vi "DriveModuleControl_TravTuneKsKv.vi"(8 "error in":errorcluster, 9 "Actual State":T1={"Speed"=0.0, "Angle"={"VALUE"=0.0, "COS"=1.0, "SIN"=0.0}} {"Angle"."SIN" format="%13.4f"; "Angle"."COS" format="%13.4f"; "Angle"."VALUE" format="%13.4f"}, 10 "Desired State":T1={"Speed"=0.0, "Angle"={"VALUE"=0.0, "COS"=1.0, "SIN"=0.0}} {"Angle"."SIN" format="%13.4f"; "Angle"."COS" format="%13.4f"; "Angle"."VALUE" format="%13.4f"}, 11 "ModualNamePrefix":i32) -> (0 "error out":errorcluster)   [LabVIEW 2023]
uses:
  <vilib>/Rock Robotics/WPI/ThirdParty/JAS_Junk/TrajLib/TypeDef/SWERVE_DRIVE_MODULE_STATE.ctl
  <vilib>/Rock Robotics/WPI/ThirdParty/JAS_Junk/TrajLib/TypeDef/ROTATION2D.ctl
  <vilib>/Rock Robotics/WPI/ThirdParty/JAS_Junk/TrajLib/LinearFilter_MovingAvg_Execute.vi
  <vilib>/Rock Robotics/WPI/ThirdParty/JAS_Junk/TrajLib/Rotation2d_Minus.vi
  <vilib>/Rock Robotics/WPI/ThirdParty/JAS_Junk/TrajLib/Rotation2d_GetRadians.vi
  <vilib>/Rock Robotics/WPI/ThirdParty/JAS_Junk/TrajLib/SwerveModuleState_New.vi
  <vilib>/Rock Robotics/WPI/ThirdParty/JAS_Junk/TrajLib/Rotation2d_RotateBy.vi
  <vilib>/Rock Robotics/WPI/ThirdParty/JAS_Junk/TrajLib/Rotation2d_CreateAngle.vi
  <vilib>/Rock Robotics/WPI/ThirdParty/JAS_Junk/TrajLib/SimpleMotorFF_Calculate.vi
  <vilib>/Rock Robotics/WPI/ThirdParty/JAS_Junk/TrajLib/PIDController_AtSetpoint.vi
  <vilib>/Rock Robotics/WPI/ThirdParty/JAS_Junk/TrajLib/PIDController_SetPIDF.vi
  <vilib>/Rock Robotics/WPI/ThirdParty/JAS_Junk/TrajLib/PIDController_SetDerivativeFilter.vi
  <vilib>/Rock Robotics/WPI/ThirdParty/JAS_Junk/TrajLib/PIDController_SetIntegratorRange.vi
  <vilib>/Rock Robotics/WPI/ThirdParty/JAS_Junk/TrajLib/PIDController_SetTolerancePandV.vi
  <vilib>/Rock Robotics/WPI/ThirdParty/JAS_Junk/TrajLib/PIDController_DisableContinousInput.vi
  <vilib>/Rock Robotics/WPI/ThirdParty/JAS_Junk/TrajLib/PIDController_EnableContinousInput.vi
  <vilib>/Rock Robotics/WPI/ThirdParty/JAS_Junk/TrajLib/PIDController_Reset.vi
  <vilib>/Rock Robotics/WPI/ThirdParty/JAS_Junk/TrajLib/PIDController_New.vi
  <vilib>/Rock Robotics/WPI/ThirdParty/JAS_Junk/TrajLib/PIDController_SetOutputLimits.vi
  <vilib>/Rock Robotics/WPI/ThirdParty/JAS_Junk/TrajLib/VI/PIDController_SetIntegratorZone.vi
  <vilib>/Rock Robotics/WPI/ThirdParty/JAS_Junk/TrajLib/LinearFilter_ResetToValue.vi
  <vilib>/Rock Robotics/WPI/ThirdParty/JAS_Junk/TrajLib/LinearFilter_Calculate.vi
  <vilib>/Rock Robotics/WPI/ThirdParty/JAS_Junk/TrajLib/Rotation2d_UnaryMinus.vi
  <vilib>/Rock Robotics/WPI/ThirdParty/JAS_Junk/TrajLib/Rotation2d_CreateXY.vi
  <vilib>/Rock Robotics/WPI/ThirdParty/JAS_Junk/TrajLib/PIDController_NewPeriod.vi
  <vilib>/Rock Robotics/WPI/ThirdParty/JAS_Junk/TrajLib/Util_CalcDist.vi
  <vilib>/Rock Robotics/SystemInterfaces/NetworkCommunication/NetComm_UsageReport_report.vi
  DriveGlobal.vi
  <vilib>/Rock Robotics/WPI/ThirdParty/Phoenix6/Phoenix6_Device_RefNumRegistryGet.vi
  <vilib>/Rock Robotics/WPI/MotorControl/WPI_MotorControlRefNum Registry Get.vi
  <vilib>/Rock Robotics/Network Tables/NT Write Number.vi
  <vilib>/Rock Robotics/WPI/ThirdParty/JAS_Junk/TrajLib/LinearFilter_MovingAverage.vi
  <vilib>/Utility/semaphor.llb/Obtain Semaphore Reference.vi
  <vilib>/Rock Robotics/WPI/ThirdParty/JAS_Junk/TrajLib/Timer_Reset.vi
  DriveTuningGlobals.vi
  <vilib>/Rock Robotics/WPI/ThirdParty/JAS_Junk/TrajLib/Globals/Util_LibraryGlobals.vi
  <vilib>/Rock Robotics/WPI/ThirdParty/JAS_Junk/TrajLib/PIDController_AdvCalculate_FF_Sp_Pv.vi
  <vilib>/Rock Robotics/WPI/ThirdParty/JAS_Junk/TrajLib/Trajectory_Library.lvlib
  <vilib>/Rock Robotics/WPI/ThirdParty/REV Robotics/REVLib/Typedef/Spark MAX Control Type.ctl
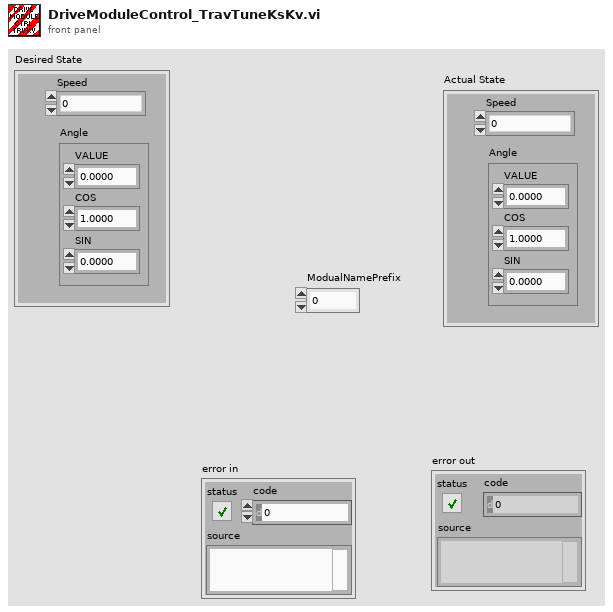
[diagram p1: front panel]
types:
  T1 = typedef "Trajectory_Library.lvlib/SWERVE_DRIVE_MODULE_STATE.ctl" = cluster{"Speed":dbl, "Angle":T2}
  T2 = typedef "Trajectory_Library.lvlib/ROTATION2D.ctl" = cluster{"VALUE":dbl, "COS":dbl, "SIN":dbl}
  T3 = typedef "Spark MAX Control Type.ctl" = enum16{"Percent VBus", "Voltage", "Velocity", "Position", "Smart Motion", "Current", "Smart Velocity", "MAXMotion Position", "MAXMotion Velocity"}
  T4 = typedef "WPI_MotorControlDeviceRef.ctl" = cluster{"DeviceStatus":errorcluster, "Type":T5, "PWM":cluster{"PWM Channel":T6, "DeadBand":T7}, "CAN":cluster{"Device Number":u8, "SetOutput VI Ref":variant, "GetOutput VI Ref":variant, "Enable VI Ref":variant, "Disable VI Ref":variant, "Data":variant}, "Invert":bool, "DIO PWM":cluster{"PWM \"Enable\" Channel":T6, "DIOChannel":T8, "PWM Rate":dbl}}
  T5 = typedef "WPI_MotorControlType.ctl" = enum16{"PWM", "CAN", "DIO PWM"}
  T6 = typedef "FPGA_DIOPWMChannel.ctl" = enum8{"PWM 0", "PWM 1", "PWM 2", "PWM 3", "PWM 4", "PWM 5", "PWM 6", "PWM 7", "PWM 8", "PWM 9", "PWM MXP 0", "PWM MXP 1", "PWM MXP 2", "PWM MXP 3", "PWM MXP 4", "PWM MXP 5", "PWM MXP 6", "PWM MXP 7", "PWM MXP 8", "PWM MXP 9", "Invalid"}
  T7 = typedef "WPI_PWMDeadband.ctl" = cluster{"Name":string, "maxPositivePwm":i32, "minPositivePwm":i32, "centerPwm":i32, "maxNegativePwm":i32, "minNegativePwm":i32, "angularRange":u16}
  T8 = typedef "FPGA_DIOChannel.ctl" = enum8{"DIO 0", "DIO 1", "DIO 2", "DIO 3", "DIO 4", "DIO 5", "DIO 6", "DIO 7", "DIO 8", "DIO 9", "DIO MXP 0", "DIO MXP 1", "DIO MXP 2", "DIO MXP 3", "DIO MXP 4", "DIO MXP 5", "DIO MXP 6", "DIO MXP 7", "DIO MXP 8", "DIO MXP 9", "DIO MXP 10", "DIO MXP 11", "DIO MXP 12", "DIO MXP 13", "DIO MXP 14", "DIO MXP 15", "SPI Port CS1", "SPI Port CS2", "SPI Port CS3", "SPI Port MISO", "SPI Port MOSI", "Invalid"}
  T9 = typedef "Trajectory_Library.lvlib/TIMER.ctl" = cluster{"StartTime":dbl, "Accumulated TIme":dbl, "Running":bool, "semaphore":T10}
  T10 = typedef "Semaphore RefNum" = refnum<k1>
  T11 = typedef "Trajectory_Library.lvlib/SIMPLE_MOTOR_FF.ctl" = cluster{"Ks":dbl, "Kv":dbl, "Ka":dbl, "KnInv":dbl}
  T12 = typedef "Trajectory_Library.lvlib/PID_ADV_LIMITS.ctl" = cluster{"MaxInput":dbl, "MinInput":dbl, "Continuous":bool, "MaxOutput":dbl, "MinOutput":dbl}
  T13 = typedef "Trajectory_Library.lvlib/PID_ADV_TUNING.ctl" = cluster{"Kf":dbl, "Kp":dbl, "Ki":dbl, "Kd":dbl, "MaximumIntegral":dbl, "MinimumIntegral":dbl, "Filter Derivative":bool, "IntegralZone":dbl}
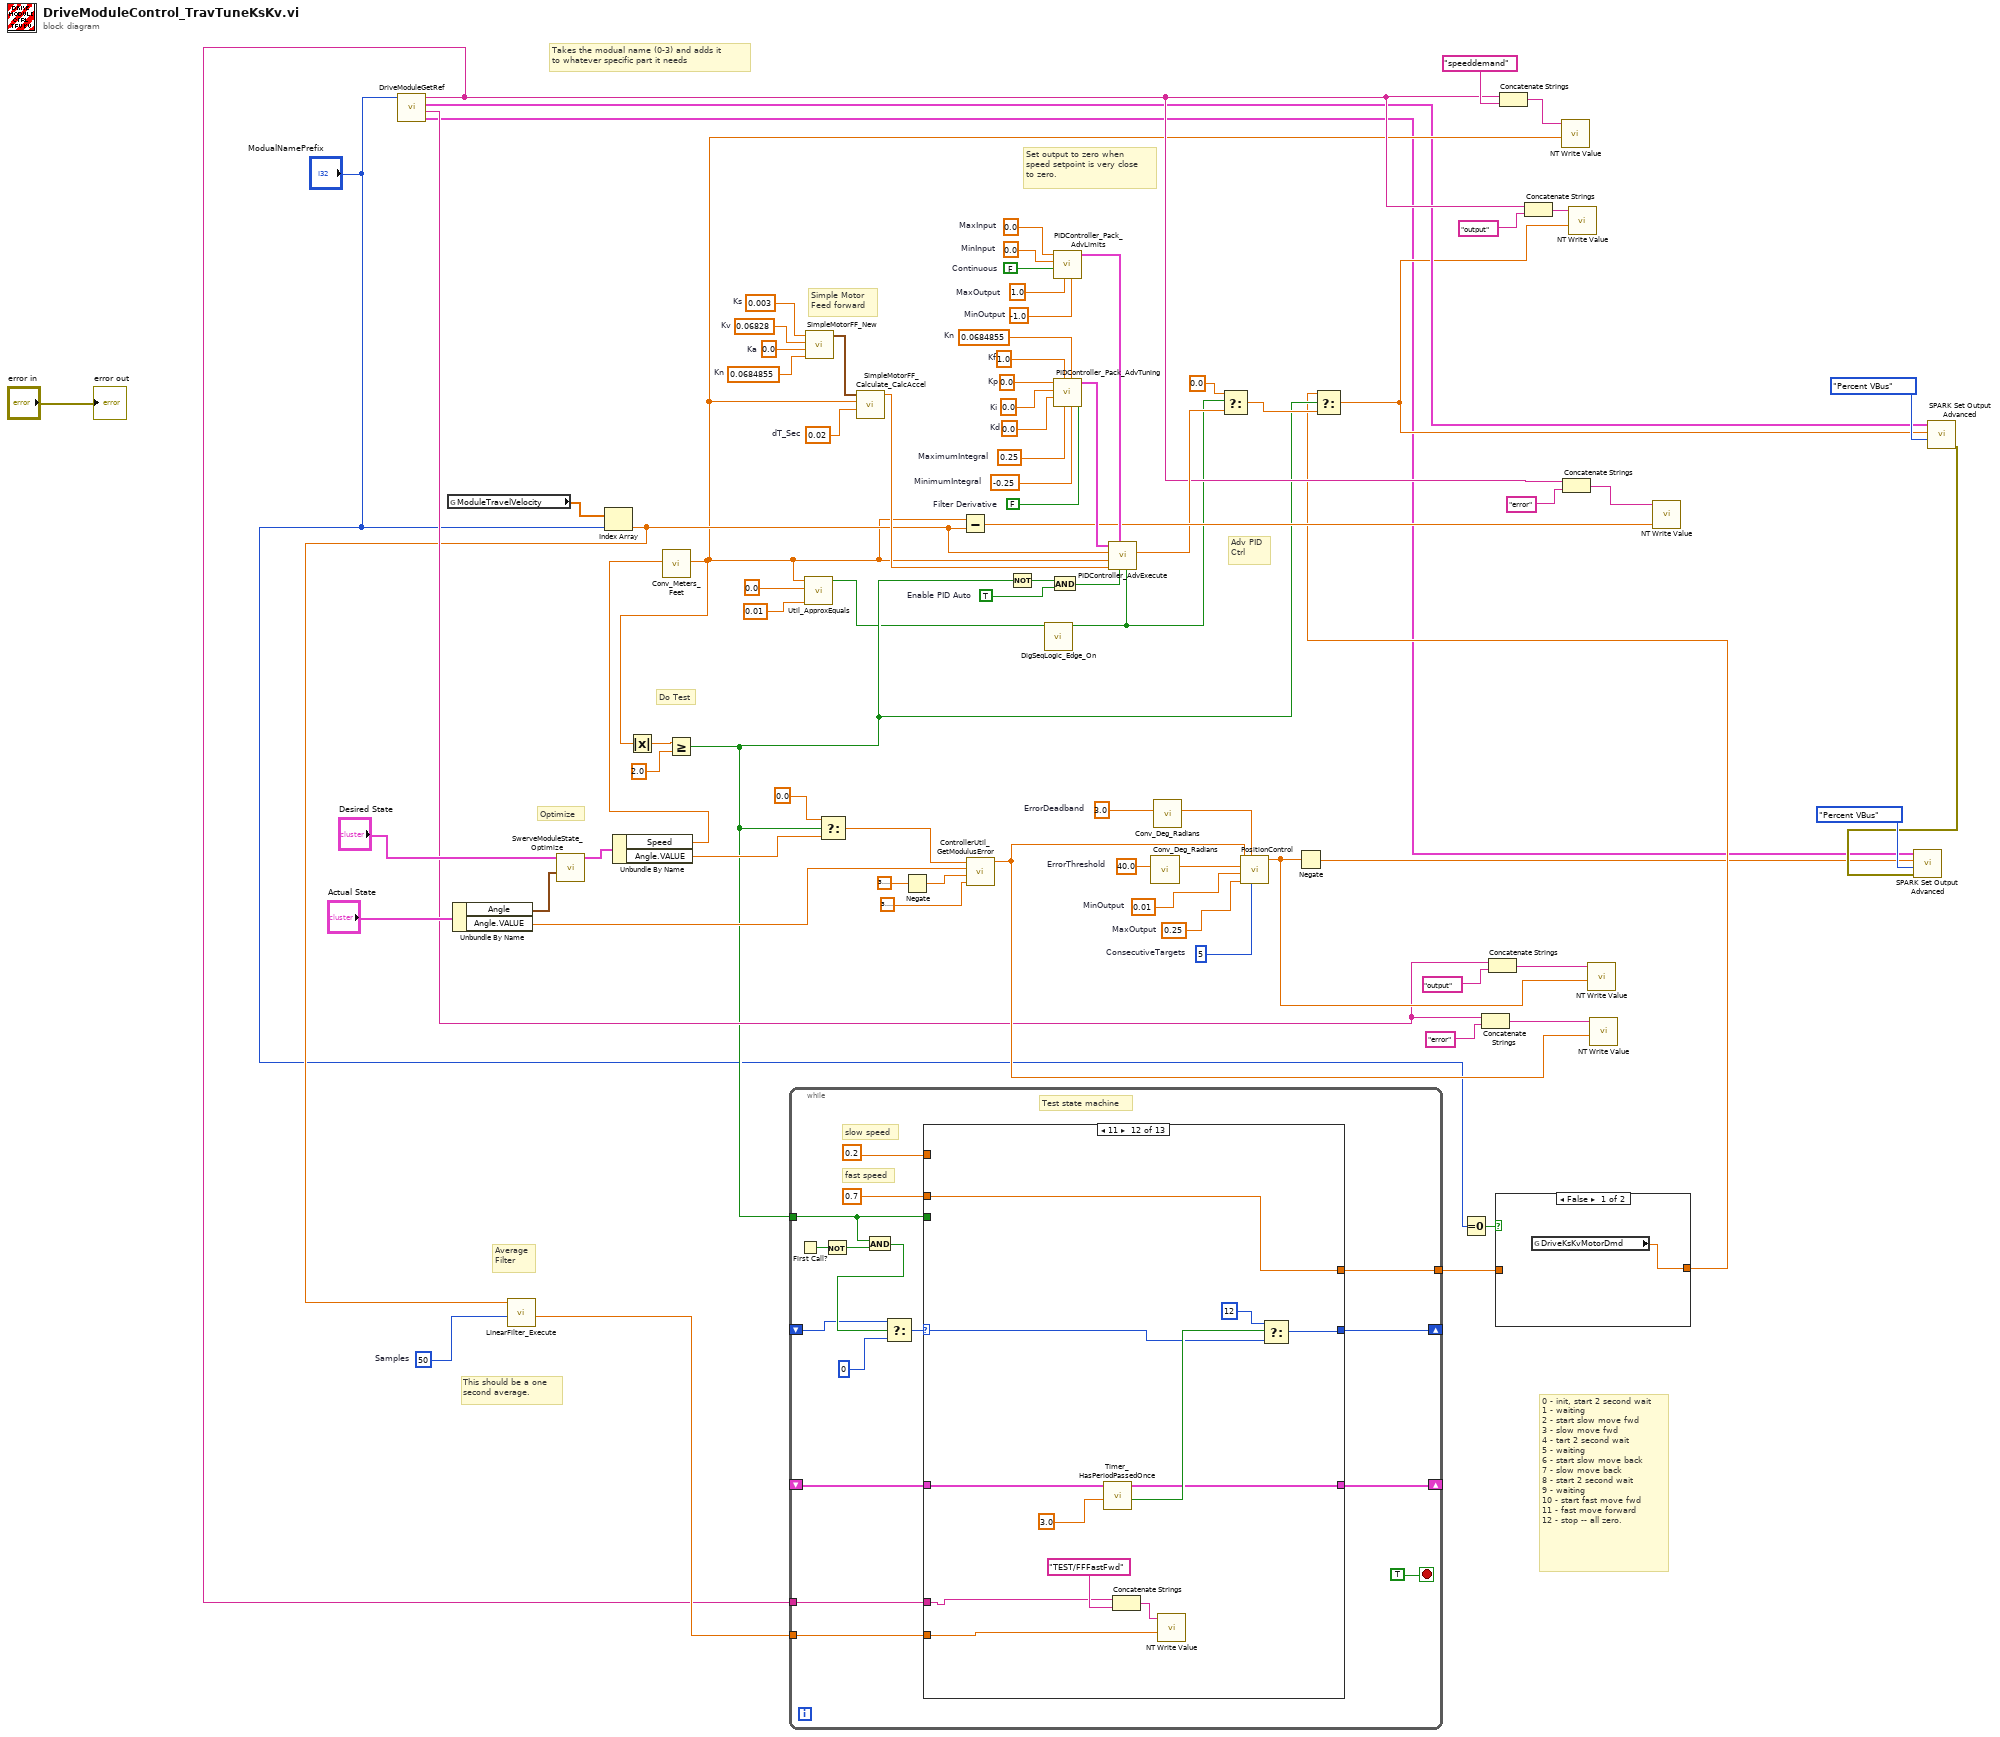
[diagram p0: block diagram]
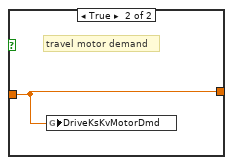
[diagram p2: hidden frame]
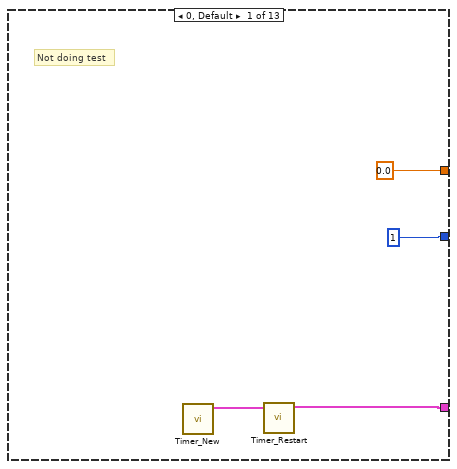
[diagram p3: hidden frame]
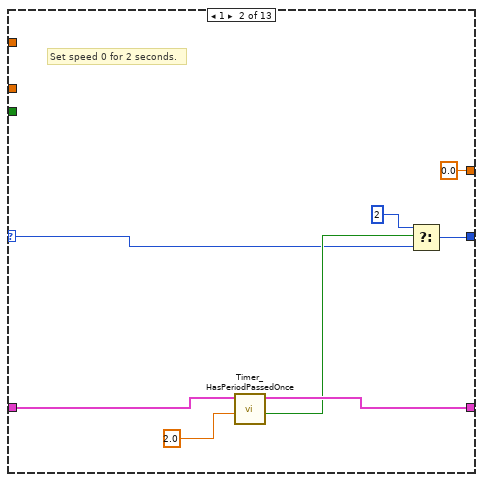
[diagram p4: hidden frame]
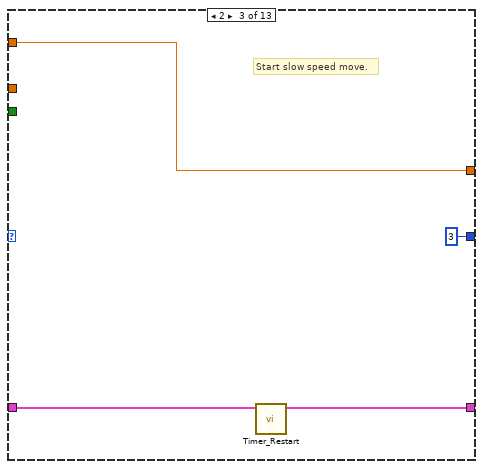
[diagram p5: hidden frame]
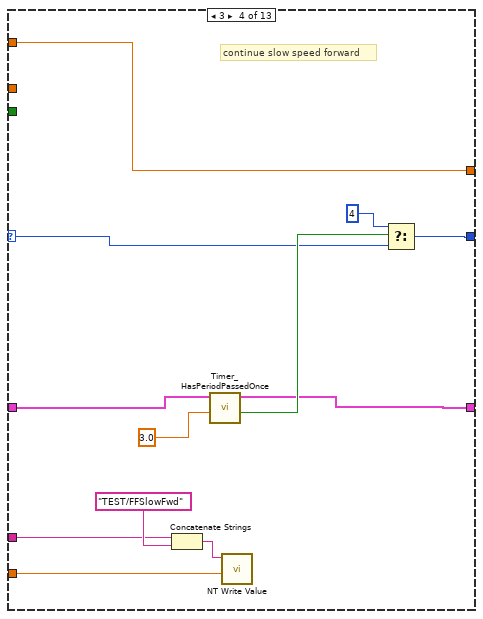
[diagram p6: hidden frame]
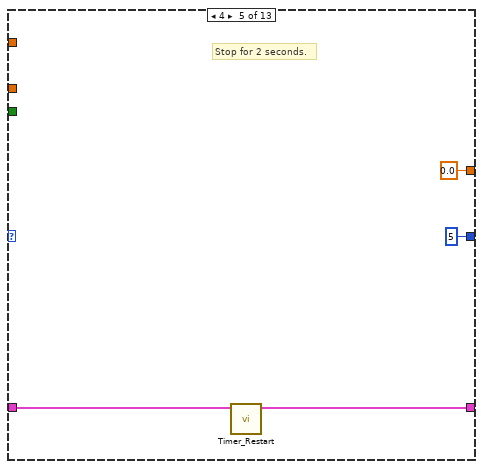
[diagram p7: hidden frame]
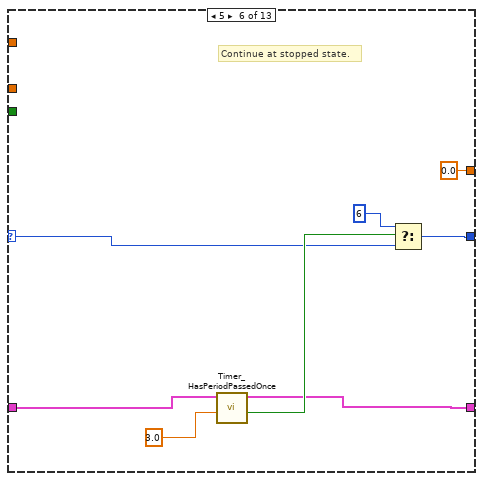
[diagram p8: hidden frame]
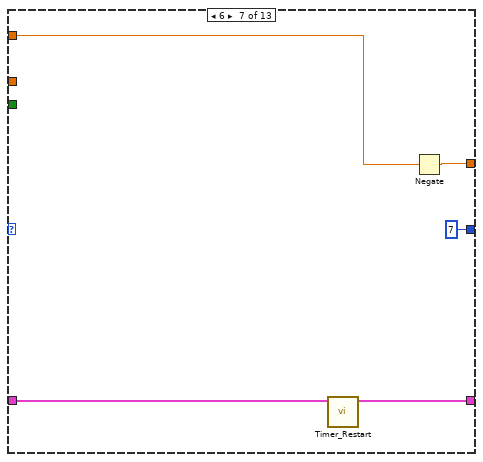
[diagram p9: hidden frame]
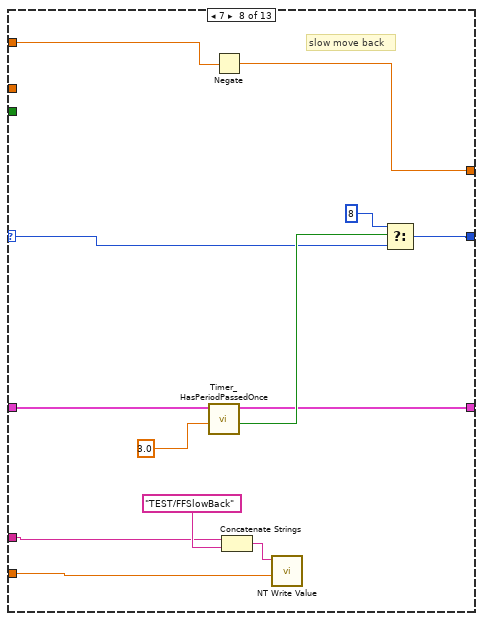
[diagram p10: hidden frame]
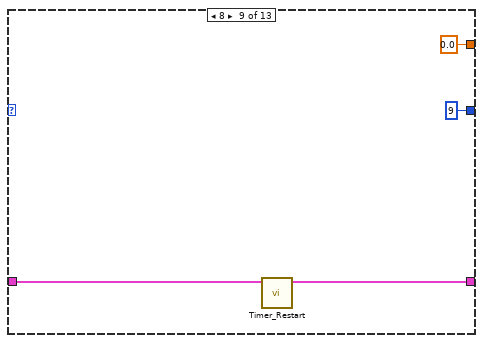
[diagram p11: hidden frame]
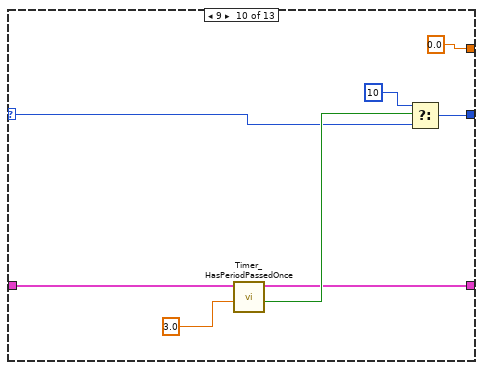
[diagram p12: hidden frame]
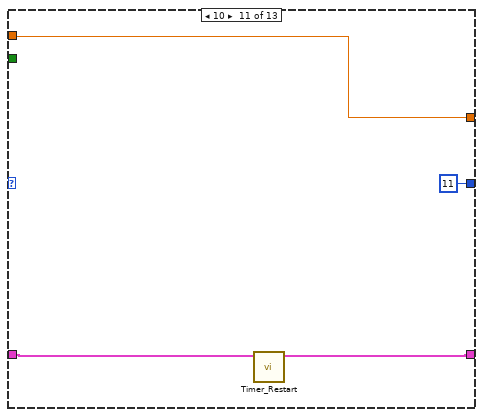
[diagram p13: hidden frame]
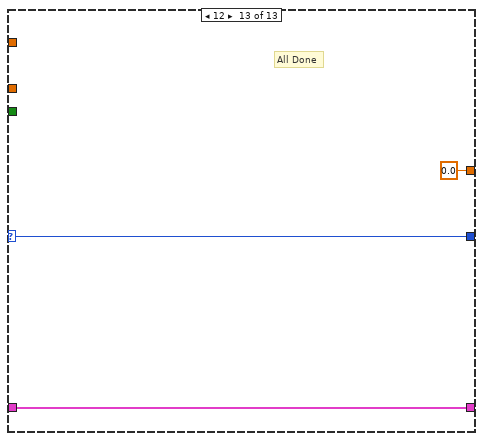
[diagram p14: hidden frame]
diagram:
  w15 = 50  # Samples
  w29 = TRUE  # Enable PID Auto
  w38 = 0.0684855  # Kn
  w54 = 0.0  # Kp
  w53 = 0.0  # Ki
  w52 = 0.0  # Kd
  w51 = 1.0  # Kf
  w50 = 0.25  # MaximumIntegral
  w49 = -0.25  # MinimumIntegral
  w48 = FALSE  # Filter Derivative
  w46 = 0.0  # MinInput
  w45 = FALSE  # Continuous
  w44 = 1.0  # MaxOutput
  w47 = -1.0  # MinOutput
  w43 = 0.0  # MaxInput
  w60 = 0.0684855  # Kn
  w59 = 0.02  # dT_Sec
  w57 = 0.003  # Ks
  w56 = 0.06828  # Kv
  w55 = 0.0  # Ka
  w69 = 5  # ConsecutiveTargets
  w66 = 0.25  # MaxOutput
  w70 = 0.01  # MinOutput
  w63 = 40.0  # ErrorThreshold
  w65 = 3.0  # ErrorDeadband
  # "This should be a one\nsecond average."
  # "Average\nFilter"
  # "0 - init, start 2 second wait\n1 - waiting\n2 - start slow move fwd\n3 - slow move fwd\n4 - tart 2 second wait\n5 - waiting\n6 - start slow move back\n7 - slow move back\n8 - start 2 second wait\n9 - waiting\n10 - start fast move fwd\n11 - fast move forward\n12 - stop -- all zero."
  # "Do Test"
  # "Optimize"
  # "Set output to zero when\nspeed setpoint is very close\nto zero."
  # "Adv PID\nCtrl"
  # "Simple Motor\nFeed forward"
  # "Takes the modual name (0-3) and adds it \nto whatever specific part it needs"
  n1 = call "DriveModuleGetRef.vi"("ModualNamePrefix"="ModualNamePrefix") -> ("SpinMot"=w2:T4, "SpinStr"=w34:string, "TravMot"=w4:T4, "TravStr"=w17:string)  [unwired: 5 in, 2 out]
  n2 = global read "DriveGlobal.vi" "ModuleTravelVelocity"() -> (w39:dbl[])
  n3 = Unbundle By Name("Actual State") -> ("Angle"=w76:T2, "Angle.VALUE"=w73:dbl)
  n4 = call <vilib>:"SwerveModuleState_Optimize.vi"("CurrentAngle"=w76, "Desired State"="Desired State") -> ("out SWERVE_DRIVE_MODULE_STATE"=w74:T1)  [unwired: 9 in]
  n5 = Index Array(array=w39, index="ModualNamePrefix") -> (element=w19:dbl)
  n6 = call-poly <vilib>:"LinearFilter_Execute.vi"("Samples"=w15, "Input"=w19) -> ("Output"=w18:dbl)  [unwired: 9 in]
  n7 = Unbundle By Name(w74) -> ("Speed"=w26:dbl, "Angle.VALUE"=w23:dbl)
  n8 = call <vilib>:"Conv_Meters_Feet.vi"("Meters"=w26) -> ("Feet"=w10:dbl)  [unwired: 10 in]
  n9 = Absolute Value(x=w10) -> (abs(x)=w25:dbl)
  n10 = Greater Or Equal?(x=w25, y=2.0) -> (x >= y?=w16:bool)
  n11 = while {
    shift-right: [w101] -> _
    shift-left: _ -> [w93]
    shift-right: [w100] -> _
    shift-left: _ -> [w91]
    tunnel: w16 -> [w95]
    tunnel: [w92] -> w14
    tunnel: w18 -> [w88]
    tunnel: w17 -> [w87]
    stop <- TRUE stop-if-true
    # "fast speed"
    # "slow speed"
    # "Test state machine"
    n12 = First Call?() -> (First Call?: T/F=w97:bool)
    n13 = Not(x=w97) -> (.not. x?=w96:bool)
    n14 = And(x=w95, y=w96) -> (x .and. y?=w94:bool)
    n15 = Select(t=w93, s=w94, f=0 ("t")) -> (s? t:f=w99:i32)
    n16 = case shown="11" w99 {
      selector: w99 -> [_ w109 _ w126 _ w138 _ w154 _ w165 _ w181 w190]
      tunnel: [1 w108 3 ("t") w127 5 ("t") w139 7 ("t") w155 9 ("t") w169 11 ("t") w184 w190] -> w101
      tunnel: [w105 w112 w116 w124 w132 w136 w147 w152 w162 w167 w173 w182 w189] -> w100
      tunnel: w95 -> [_ _ _ _ _ _ _ _ _ _ _ _ _]
      tunnel: [0.0 0.0 w115 w123 0.0 0.0 w144 w159 0.0 0.0 w176 w188 0.0] -> w92
      tunnel: w91 -> [_ w113 w117 w125 w133 w137 w146 w153 w161 w168 w174 w183 w189]
      tunnel: 0.2 -> [_ _ w115 w123 _ _ w143 w160 _ _ _ _ _]
      tunnel: 0.7 -> [_ _ _ _ _ _ _ _ _ _ w176 w188 _]
      tunnel: w88 -> [_ _ _ w122 _ _ _ w148 _ _ _ w177 _]
      tunnel: w87 -> [_ _ _ w119 _ _ _ w149 _ _ _ w178 _]
      frame 0, Default {
        # "Not doing test"
        n17 = call <vilib>:"Timer_New.vi"() -> ("TIMER"=w106:T9)  [unwired: 11 in]
        n18 = call <vilib>:"Timer_Restart.vi"("in Timer"=w106) -> ("out Timer"=w105:T9)  [unwired: 10 in]
      }
      frame 1 {
        # "Set speed 0 for 2 seconds."
        n19 = call <vilib>:"Timer_HasPeriodPassedOnce.vi"("Period"=2.0, "in Timer"=w113) -> ("Expired"=w110:bool, "out Timer"=w112:T9)  [unwired: 7 in, 1 out]
        n20 = Select(t=2, s=w110, f=w109) -> (s? t:f=w108:i32)
      }
      frame 2 {
        # "Start slow speed move."
        n21 = call <vilib>:"Timer_Restart.vi"("in Timer"=w117) -> ("out Timer"=w116:T9)  [unwired: 10 in]
      }
      frame 3 {
        # "continue slow speed forward"
        n22 = Concatenate Strings(w119, "TEST/FFSlowFwd" ("refnum name")) -> (w120:string)
        n23 = call <vilib>:"Timer_HasPeriodPassedOnce.vi"("Period"=3.0, "in Timer"=w125) -> ("Expired"=w129:bool, "out Timer"=w124:T9)  [unwired: 7 in, 1 out]
        n24 = call-poly <vilib>:"NT Write Value.vi"("value"=w122, "name"=w120) -> ()  [unwired: 9 in, 1 out]
        n25 = Select(t=4, s=w129, f=w126) -> (s? t:f=w127:i32)
      }
      frame 4 {
        # "Stop for 2 seconds."
        n26 = call <vilib>:"Timer_Restart.vi"("in Timer"=w133) -> ("out Timer"=w132:T9)  [unwired: 10 in]
      }
      frame 5 {
        # "Continue at stopped state."
        n27 = call <vilib>:"Timer_HasPeriodPassedOnce.vi"("Period"=3.0, "in Timer"=w137) -> ("Expired"=w141:bool, "out Timer"=w136:T9)  [unwired: 7 in, 1 out]
        n28 = Select(t=6, s=w141, f=w138) -> (s? t:f=w139:i32)
      }
      frame 6 {
        n29 = call <vilib>:"Timer_Restart.vi"("in Timer"=w146) -> ("out Timer"=w147:T9)  [unwired: 10 in]
        n30 = Negate(x=w143) -> (-x=w144:dbl)
      }
      frame 7 {
        # "slow move back"
        n31 = call <vilib>:"Timer_HasPeriodPassedOnce.vi"("Period"=3.0, "in Timer"=w153) -> ("Expired"=w157:bool, "out Timer"=w152:T9)  [unwired: 7 in, 1 out]
        n32 = Negate(x=w160) -> (-x=w159:dbl)
        n33 = Concatenate Strings(w149, "TEST/FFSlowBack" ("refnum name")) -> (w150:string)
        n34 = call-poly <vilib>:"NT Write Value.vi"("value"=w148, "name"=w150) -> ()  [unwired: 9 in, 1 out]
        n35 = Select(t=8, s=w157, f=w154) -> (s? t:f=w155:i32)
      }
      frame 8 {
        n36 = call <vilib>:"Timer_Restart.vi"("in Timer"=w161) -> ("out Timer"=w162:T9)  [unwired: 10 in]
      }
      frame 9 {
        n37 = call <vilib>:"Timer_HasPeriodPassedOnce.vi"("Period"=3.0, "in Timer"=w168) -> ("Expired"=w171:bool, "out Timer"=w167:T9)  [unwired: 7 in, 1 out]
        n38 = Select(t=10, s=w171, f=w165) -> (s? t:f=w169:i32)
      }
      frame 10 {
        n39 = call <vilib>:"Timer_Restart.vi"("in Timer"=w174) -> ("out Timer"=w173:T9)  [unwired: 10 in]
      }
      frame 11 {
        n40 = call <vilib>:"Timer_HasPeriodPassedOnce.vi"("Period"=3.0, "in Timer"=w183) -> ("Expired"=w186:bool, "out Timer"=w182:T9)  [unwired: 7 in, 1 out]
        n41 = Concatenate Strings(w178, "TEST/FFFastFwd" ("refnum name")) -> (w179:string)
        n42 = call-poly <vilib>:"NT Write Value.vi"("value"=w177, "name"=w179) -> ()  [unwired: 9 in, 1 out]
        n43 = Select(t=12, s=w186, f=w181) -> (s? t:f=w184:i32)
      }
      frame 12 {
        # "All Done"
      }
    }
  }
  n44 = call <vilib>:"Util_ApproxEquals.vi"("Tolerance"=0.01, "Value 2"=0.0, "Value 1"=w10) -> ("ApproxEquals"=w9:bool)  [unwired: 8 in]
  n45 = call <vilib>:"SimpleMotorFF_New.vi"("Kn"=w60, "Ka"=w55, "Kv"=w56, "Ks"=w57) -> ("SIMPLE_MOTOR_FF"=w58:T11)  [unwired: 7 in]
  n46 = Select(t=0.0, s=w16, f=w23) -> (s? t:f=w20:dbl)
  n47 = call <vilib>:"SimpleMotorFF_Calculate_CalcAccel.vi"("dT_Sec"=w59, "VelSp"=w10, "SIMPLE_MOTOR_FF"=w58) -> ("FeedForward"=w40:dbl)  [unwired: 8 in]
  n48 = Negate(x=3.141592653589793) -> (-x=w75:dbl)
  n49 = Subtract(x=w10, y=w19) -> (x-y=w35:dbl)
  n50 = call <vilib>:"ControllerUtil_GetModulusError.vi"("Maximum_Input"=3.141592653589793, "Minimum_Input"=w75, "Measurerment(PV)"=w73, "Reference(SP)"=w20) -> ("Error"=w67:dbl)  [unwired: 7 in]
  n51 = Not(x=w16) -> (.not. x?=w30:bool)
  n52 = call <vilib>:"DigSeqLogic_Edge_On.vi"("Input"=w9) -> ("On Edge"=w8:bool)  [unwired: 10 in]
  n53 = And(x=w30, y=w29) -> (x .and. y?=w31:bool)
  n54 = call <vilib>:"PIDController_Pack_AdvLimits.vi"("MinOutput"=w47, "MaxOutput"=w44, "Continuous"=w45, "MinInput"=w46, "MaxInput"=w43) -> ("Adv PID Limits"=w41:T12)  [unwired: 6 in]
  n55 = call <vilib>:"PIDController_Pack_AdvTuning.vi"("Filter Derivative"=w48, "MinimumIntegral"=w49, "Kn"=w38, "MaximumIntegral"=w50, "Kf"=w51, "Kd"=w52, "Ki"=w53, "Kp"=w54) -> ("Adv PID Tuning"=w42:T13)  [unwired: 3 in]
  n56 = call <vilib>:"PIDController_AdvExecute.vi"("Reset"=w8, "Auto"=w31, "Adv PID Limits"=w41, "FF-FeedForward"=w40, "SP-SetPoint"=w10, "PV-Measurement"=w19, "Adv PID Tuning"=w42) -> ("CO-ControlOutput"=w28:dbl)  [unwired: 2 in, 2 out]
  n57 = call <vilib>:"Conv_Deg_Radians.vi"("Degress"=w63) -> ("Radians"=w62:dbl)  [unwired: 10 in]
  n58 = call <vilib>:"Conv_Deg_Radians.vi"("Degress"=w65) -> ("Radians"=w64:dbl)  [unwired: 10 in]
  n59 = Select(t=0.0, s=w8, f=w28) -> (s? t:f=w21:dbl)
  n60 = call "PositionControl.vi"("ConsecutiveTargets"=w69, "ErrorDeadband"=w64, "MaxOutput"=w66, "MinOutput"=w70, "ErrorThreshold"=w62, "Error"=w67) -> ("OutputValue"=w61:dbl)  [unwired: 3 in, 2 out]
  n61 = Negate(x=w61) -> (-x=w1:dbl)
  n62 = Equal To 0?(x="ModualNamePrefix") -> (x = 0?=w13:bool)
  n63 = Concatenate Strings(w34, "error" ("refnum name")) -> (w80:string)
  n64 = Concatenate Strings(w34, "output" ("refnum name")) -> (w68:string)
  n65 = case shown="False" w13 {
    tunnel: w14 -> [_ w193]
    tunnel: [w192 w193] -> w11
    frame False {
      n66 = global read "DriveTuningGlobals.vi" "DriveKsKvMotorDmd"() -> (w192:dbl)
    }
    frame True {
      # "travel motor demand"
      n67 = global write "DriveTuningGlobals.vi" "DriveKsKvMotorDmd"(w193) -> ()
    }
  }
  n68 = Select(t=w11, s=w16, f=w21) -> (s? t:f=w3:dbl)
  n69 = Concatenate Strings(w17, "speeddemand" ("refnum name")) -> (w84:string)
  n70 = Concatenate Strings(w17, "output" ("refnum name")) -> (w82:string)
  n71 = call-poly <vilib>:"NT Write Value.vi"("value"=w10, "name"=w84) -> ()  [unwired: 9 in, 1 out]
  n72 = Concatenate Strings(w17, "error" ("refnum name")) -> (w36:string)
  n73 = call-poly <vilib>:"NT Write Value.vi"("value"=w3, "name"=w82) -> ()  [unwired: 9 in, 1 out]
  n74 = call-poly <vilib>:"NT Write Value.vi"("value"=w61, "name"=w68) -> ()  [unwired: 9 in, 1 out]
  n75 = call-poly <vilib>:"NT Write Value.vi"("value"=w67, "name"=w80) -> ()  [unwired: 9 in, 1 out]
  n76 = call-poly <vilib>:"NT Write Value.vi"("value"=w35, "name"=w36) -> ()  [unwired: 9 in, 1 out]
  n77 = call <vilib>:"SPARK Set Output Advanced.vi"("Control Mode"=Spark_MAX_Control_Type."Percent VBus", "Setpoint"=w3, "MotorControlDevRef"=w4) -> ("error out"=w5:errorcluster)  [unwired: 7 in, 1 out]
  n78 = call <vilib>:"SPARK Set Output Advanced.vi"("error in (no error)"=w5, "Control Mode"=Spark_MAX_Control_Type."Percent VBus", "Setpoint"=w1, "MotorControlDevRef"=w2) -> ()  [unwired: 6 in, 2 out]
  "error out" <- "error in"
